vi "Reciev_CANATII.vi"(2 "cnd_in":u32, 3 "queue out":refnum<queue>, 4 "Config":refnum<vi>) -> (0 "Data":u8[](array[numeric]), 1 "cnt_out":u32)   [LabVIEW 2017]
uses:
  PCAN_Driver/ControlCAN.lvlib
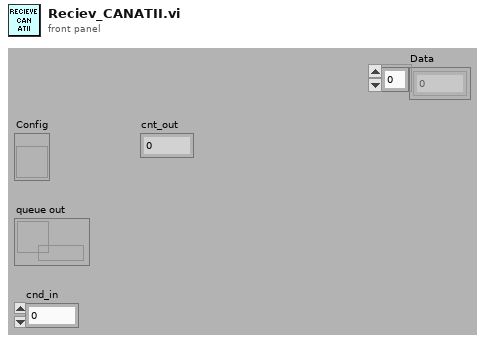
[diagram p1: front panel]
types:
  T1 = typedef "ControlCAN.lvlib/DevType.ctl" = u32
  T2 = typedef "ControlCAN.lvlib/CAN Channel.ctl" = u32
  T3 = typedef "ControlCAN.lvlib/VCI_INIT_CONFIG.ctl" = cluster{"AccCode":u32, "AccMask":u32, "InitFlag":T4, "Fliter":T5, "Timing0":u8, "Timing1":u8, "Mode":T6}
  T4 = typedef "ControlCAN.lvlib/InitFlag.ctl" = u32
  T5 = typedef "ControlCAN.lvlib/Fliter.ctl" = u8
  T6 = typedef "ControlCAN.lvlib/Mode.ctl" = u8
  T7 = cluster{"DevType":T1, "DevIndex":u32, "CanIndex":T2, "VCI_INIT_CONFIG":T3}
  T8 = typedef "ControlCAN.lvlib/VCI_CAN_OBJ.ctl" = cluster{"ID":u32, "TimeStamp":u32, "TimeFlag":u8, "SendType":u8, "RemoteFlag":u8, "ExternFlag":u8, "DataLen":u8, "Data":u8[], "Reserved":u8[]}
  T9 = cluster{"ID":u32, "MSGTYPE":u8, "LEN":u8, "aDATA":u8[]}
  T10 = cluster{"Type":enum16{"接收", "发送"}, "Channel":T2, "Time":timestamp, "VCI_CAN_OBJ":T8}[]
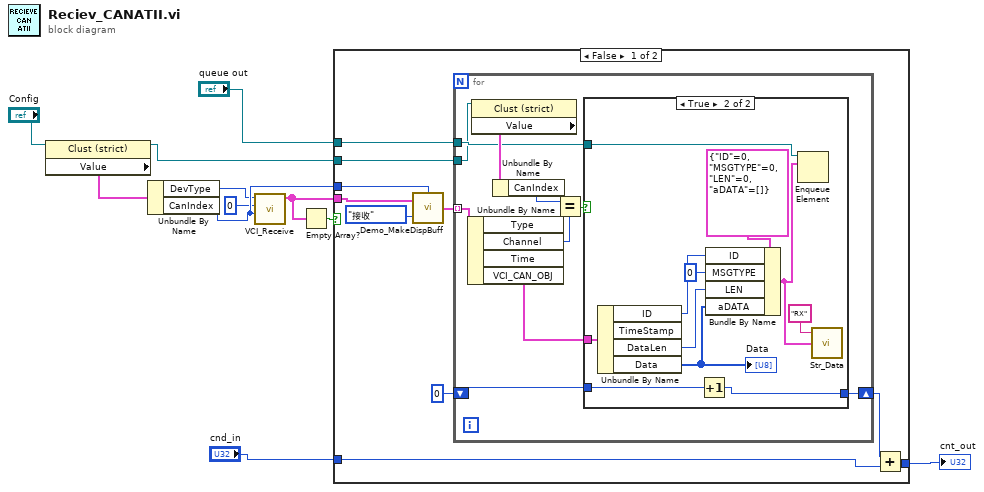
[diagram p0: block diagram]
diagram:
  n1 = property class="Clust (strict)"(reference="Config") -> (reference out=w1:refnum<vi>, "Value"=w8:T7)  [unwired: 1 in, 1 out]
  n2 = Unbundle By Name(w8) -> ("DevType"=w6:T1, "CanIndex"=w7:T2)
  n3 = call "VCI_Receive.vi"("CANIndex"=w7, "DevIndex"=u32 0, "DevType"=w6) -> ("Recieve"=w5:T8[])  [unwired: 3 in, 5 out]
  n4 = Empty Array?(array=w5) -> (empty?=w4:bool)
  n5 = case shown="False" w4 {
    tunnel: w5 -> [w19 _]
    tunnel: w7 -> [w20 _]
    tunnel: "cnd_in" -> [w15 w44]
    tunnel: [w14 w44] -> w9
    tunnel: "queue out" -> [w13 _]
    tunnel: w1 -> [w12 _]
    frame False {
      n6 = call "Demo_MakeDispBuff.vi"("Channel"=w20, "Type"=enum16{"接收", "发送"}."接收", "OBJs"=w19) -> ("Buffer"=w18:T10)
      n7 = for {
        tunnel: w18 -> [w31] mode=indexing
        tunnel: w13 -> [w23]
        shift-right: [w24] -> w16
        shift-left: u32 0 -> [w25]
        tunnel: w12 -> [w22]
        n8 = Unbundle By Name(w31) -> ("Channel"=w27:T2, "VCI_CAN_OBJ"=w30:T8)  [unwired: 2 out]
        n9 = property class="Clust (strict)"(reference=w22) -> ("Value"=w29:T7)  [unwired: 1 in, 2 out]
        n10 = Unbundle By Name(w29) -> ("CanIndex"=w28:T2)
        n11 = Equal?(x=w28, y=w27) -> (x = y?=w26:bool)
        n12 = case shown="True" w26 {
          tunnel: w23 -> [_ w36]
          tunnel: w30 -> [_ w42]
          tunnel: w25 -> [w32 w38]
          tunnel: [w32 w37] -> w24
          frame False {
          }
          frame True {
            n13 = Unbundle By Name(w42) -> ("ID"=w41:u32, "DataLen"=w40:u8, "Data"=w39:u8[])  [unwired: 1 out]
            "Data" <- w39
            n14 = Increment(x=w38) -> (x+1=w37:u32)
            n15 = Bundle By Name(cluster=T9 {"ID"=0, "MSGTYPE"=0, "LEN"=0, "aDATA"=[]} ("Msg"), "ID"=w41, "MSGTYPE"=u8 0, "LEN"=w40, "aDATA"=w39) -> (w34:T9)
            n16 = Enqueue Element(queue=w36, element=w34) -> ()  [unwired: 1 in, 4 out]
            n17 = call "Str_Data.vi"("Msg"=w34, "string"="RX") -> ()  [unwired: 1 in, 1 out]
          }
        }
      }
      n18 = Add(x=w16, y=w15) -> (x+y=w14:u32)
    }
    frame True {
    }
  }
  "cnt_out" <- w9
